vi "MAIN_green.vi"() -> ()   [LabVIEW 2011]
uses:
  <vilib>/userDefined/High Color/IMAQdx.ctl
  <vilib>/vision/driver/NI_Vision_Acquisition_Software.lvlib
  <vilib>/vision/NI_Vision_Development_Module.lvlib
panel:
  out "error out 6":errorcluster
  out "error out 5":errorcluster
  out "error out 4":errorcluster
  in  "SLM 2":enum32{"Viewer & Positioner", "Hologram Loader"}(tab)
  out "<< CGH_y\n      SLM 2":T1(plugin-control)
  in  "X position 2":dbl(slide)=1.056105610561056 scale=0.0..10.0
  in  "Fine:":dbl(slide)=2.7960526315789473 scale=0.0..10.0
  out "X 2":dbl
  in  "Fine:":dbl(slide)=4.922480620155039 scale=0.0..10.0
  in  "Y position 3":dbl(slide)=3.875968992248062 scale=0.0..10.0
  out "Y position 2":dbl
  out "String 2":string
  out "String 3":string
  out "SLM 3":T1(plugin-control)
  in  "Radio Buttons":T2(radio)=enum."Radio Selection 2"
  in  "Semi2":bool caption="Boolean"
  in  "Phase correction 2":bool
  in  "M4":bool
  in  "Holo:":dbl=1.0
  out "Ph2 2":dbl
  out "[0 255]":dbl
  out "Ph2":dbl
  in  "Phase:":dbl(slide) scale=0.0..360.0
  out "T2":dbl=100.0
  in  "Trans.:":dbl(slide)=100.0 scale=0.0..100.0
  in  "Active SLM2":bool=TRUE
  in  "SLM 1":enum32{"Viewer & Positioner", "Hologram Loader"}(tab)
  out "CGH_x >>\nSLM 1":T1(plugin-control)
  in  "Y position":dbl(slide)=3.292682926829268 scale=0.0..10.0
  in  "X position 1":dbl(slide)=8.30670926517572 scale=0.0..10.0
  in  "Fine:":dbl(slide)=7.667731629392971 scale=0.0..10.0
  in  "Fine:":dbl(slide)=0.7636363636363636 scale=0.0..10.0
  out "X position":dbl
  out "Y position 1":dbl
  out "String":string
  in  "Radio Buttons 2":T2(radio)=enum."Radio Selection 2"
  in  "Semi":bool caption="Boolean"
  in  "Phase correction":bool caption="Amplitude correction"
  in  "M4 2":bool caption="Amplitude correction"
  in  "Holo:":dbl=1.0
  out "Ph1 2":dbl
  out "[0 255]":dbl
  out "Ph1":dbl
  in  "Phase:":dbl(slide) scale=0.0..360.0
  out "T1":dbl=100.0
  in  "Trans.:":dbl(slide)=100.0 scale=0.0..100.0
  out "SLM 2":T1(plugin-control)
  in  "Active SLM1":bool=TRUE
  out "String 4":string
  in  "Parada Total":bool
  in  "Tab Control":enum32{"Laser Control", "CCD viewer"}(tab)
  in  "APTLaser":refnum<k7>(container) caption="Resume"
  in  "LaserON":bool
  in  "Set Current at:":sgl=70.0 caption="mA"
  out "Color Box":u32(colorbox)
  out "Power":dbl(knob) caption="mW" scale=0.0..16.0
  in  "Save":bool
  in  "Focused":bool
  out "Image":T1(plugin-control)
  out "Histograph":T3(graph)={"Starting Value"=-32768.0, "Incremental Value"=1.0, "Histogram"=array[65536 elements]}
  out "# Sat. Pixels":sgl(slide) scale=0.0..5000.0
  out "error out 3":errorcluster
  out "error out 2":errorcluster
  out "error out":errorcluster
  out "path":path
  out "selected path 2":path
  out "selected path":path
  # "Arbitrary value settings:"
  # "For gray levels ->"
  # "%"
  # "º"
  # "\\pi rad"
  # "Arbitrary value settings:"
  # "For gray levels ->"
  # "%"
  # "º"
  # "\\pi rad"
  # "Paraxial"
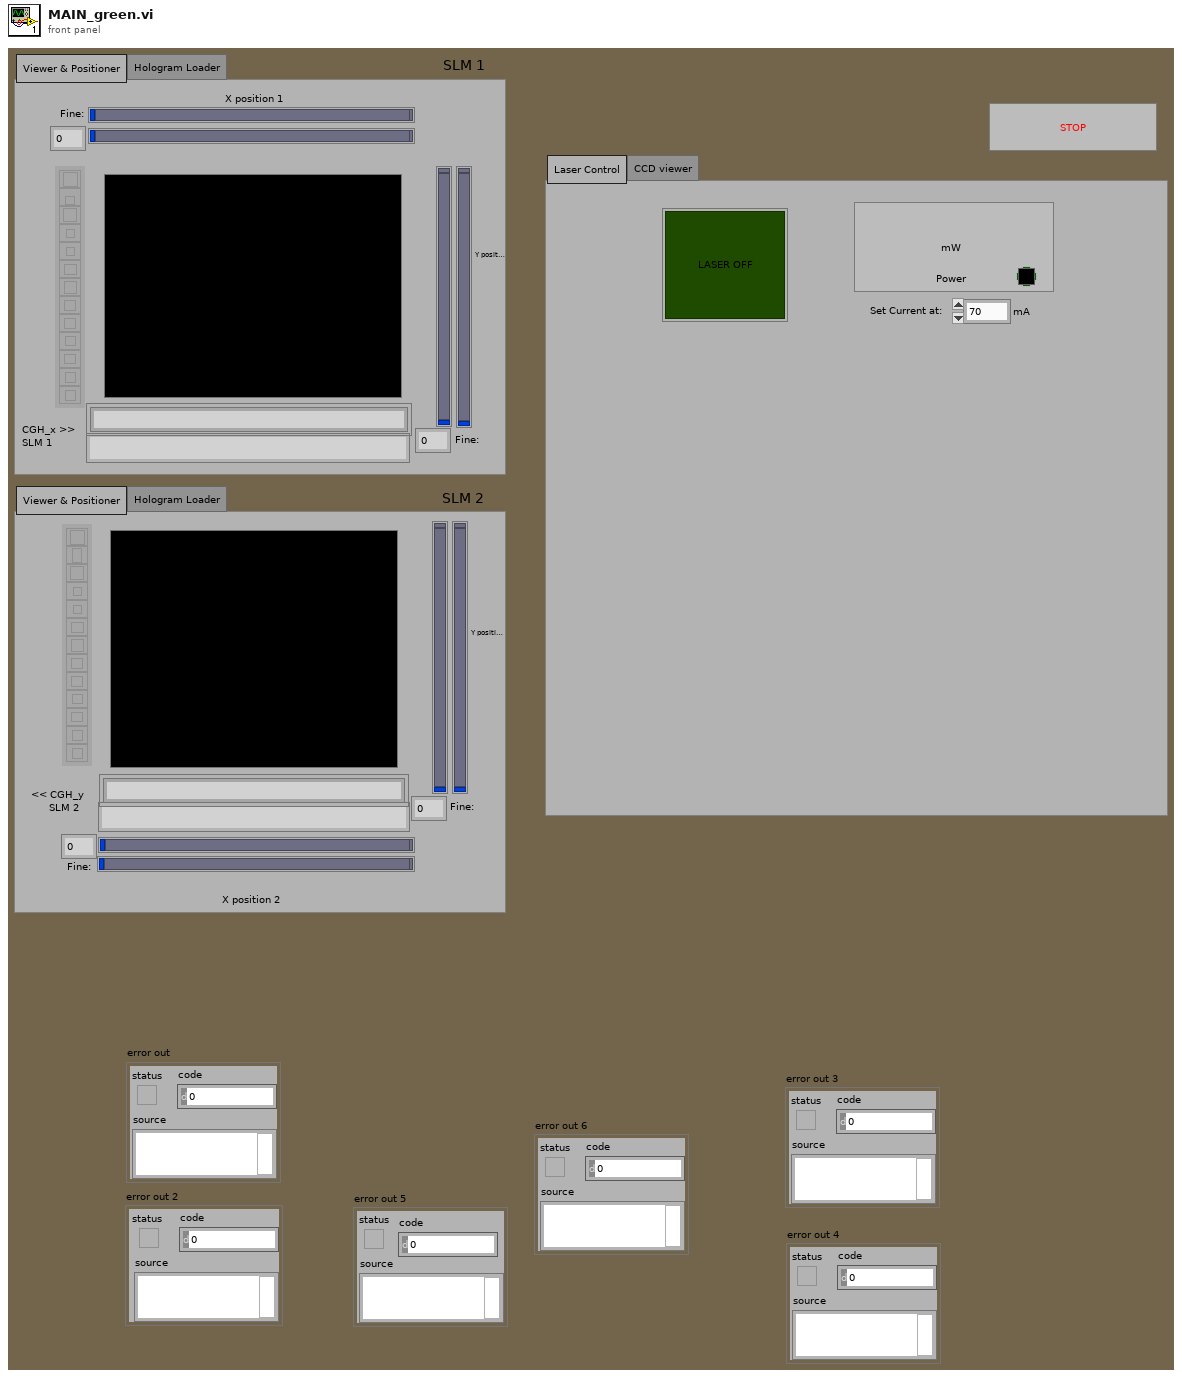
[diagram p1: front panel]
types:
  T1 = typedef "IMAQ Image.ctl" = refnum<image>
  T2 = enum32{"Radio Selection 1", "Radio Selection 2", "Radio Selection 3", "Radio Selection 4", "Radio Selection 5", "Radio Selection 6", "Radio Selection 7"}
  T3 = cluster{"Starting Value":sgl, "Incremental Value":sgl, "Histogram":u32[]}
  T4 = typedef "IMAQdx.ctl" = refnum<k21>
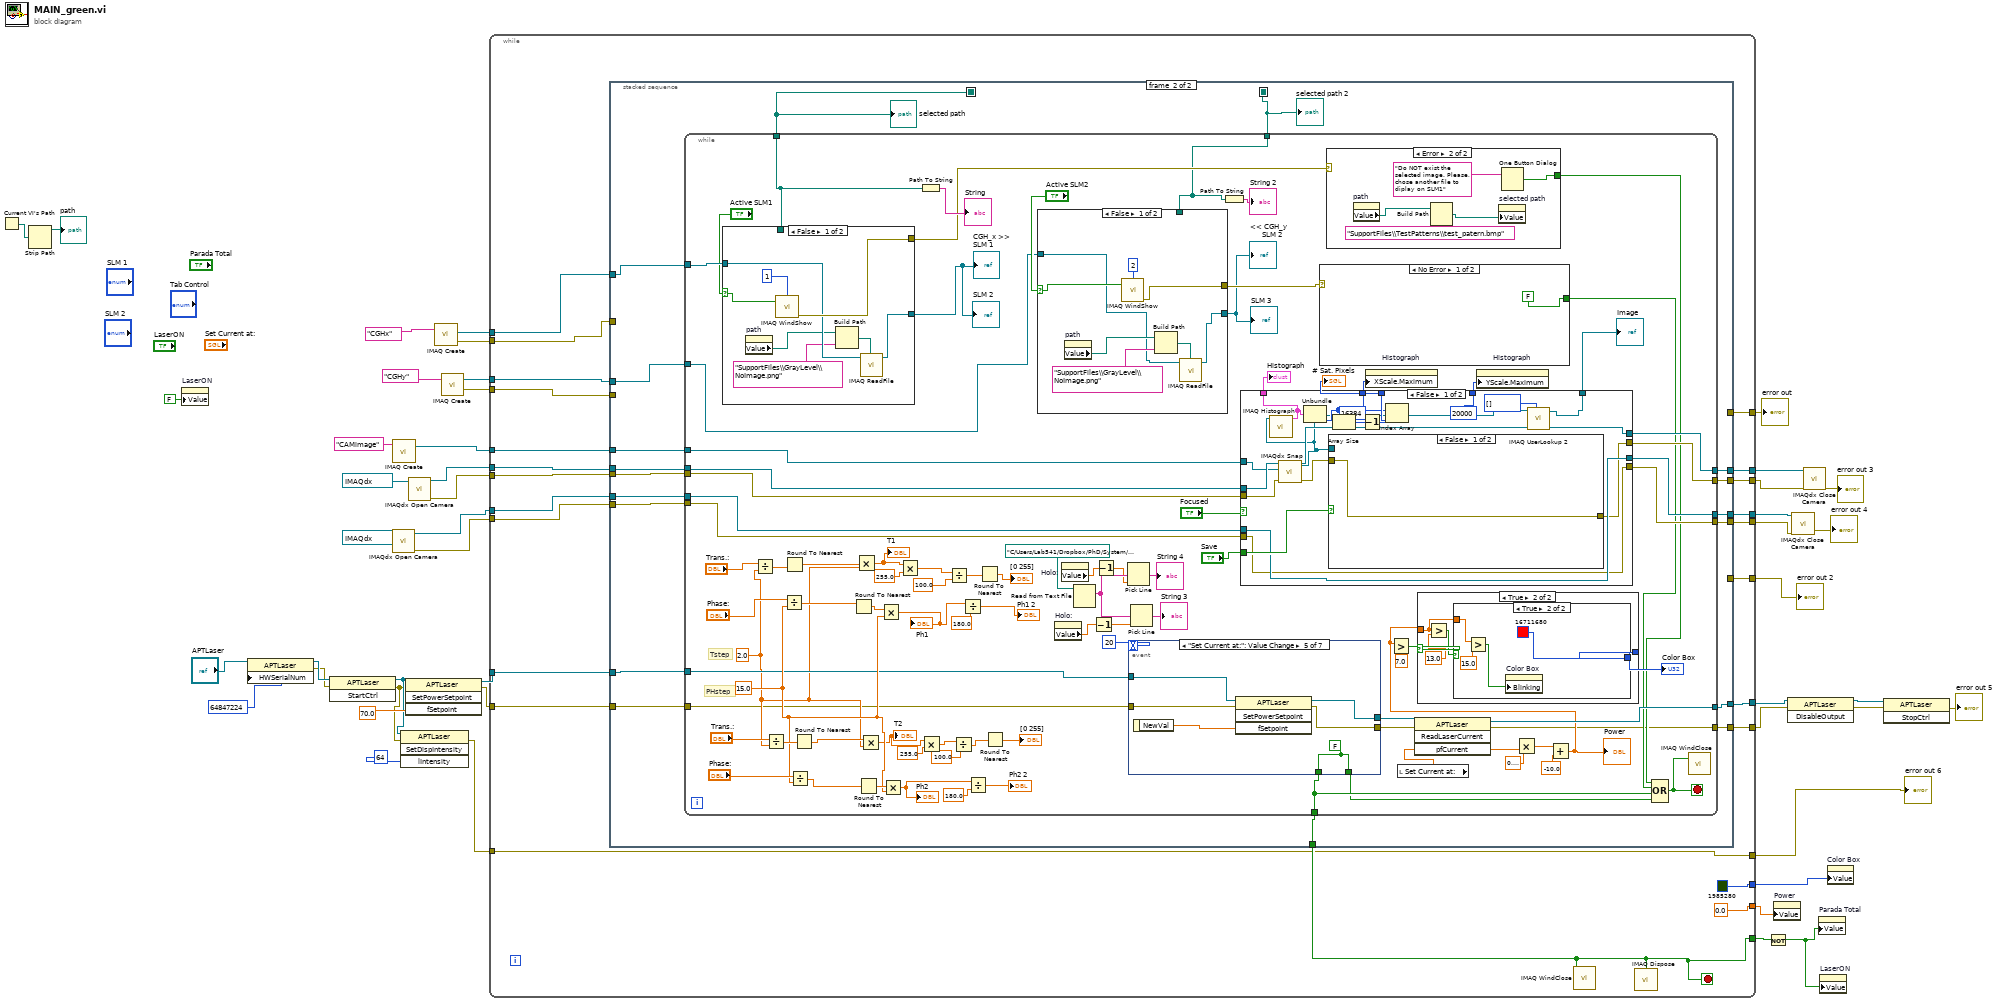
[diagram p0: block diagram]
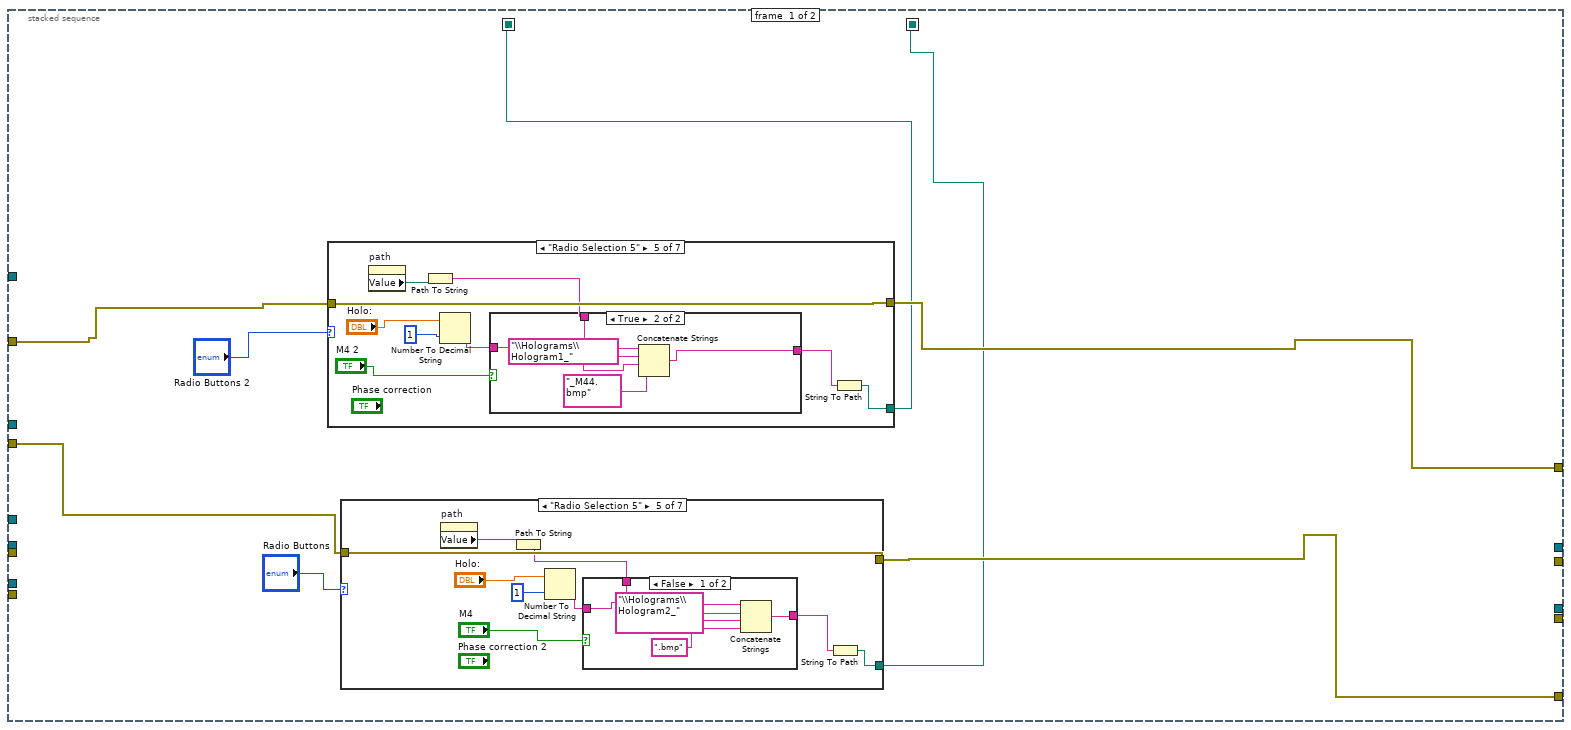
[diagram p2: hidden frame]
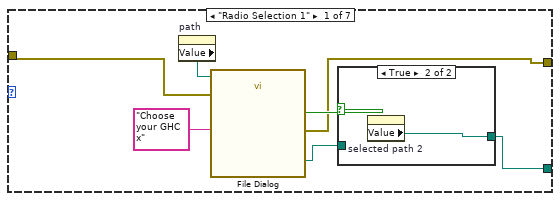
[diagram p3: hidden frame]
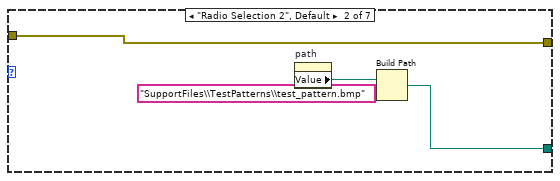
[diagram p5: hidden frame]
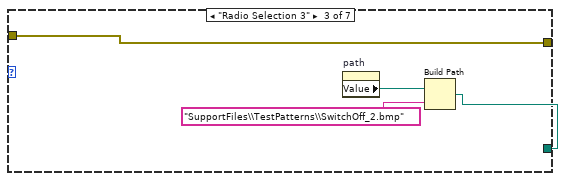
[diagram p6: hidden frame]
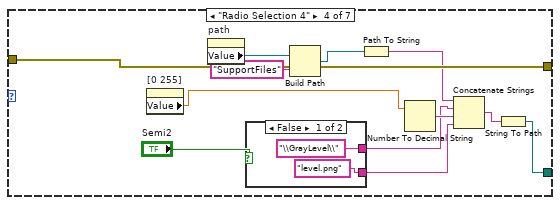
[diagram p7: hidden frame]
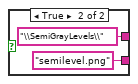
[diagram p8: hidden frame]
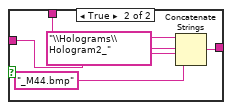
[diagram p9: hidden frame]
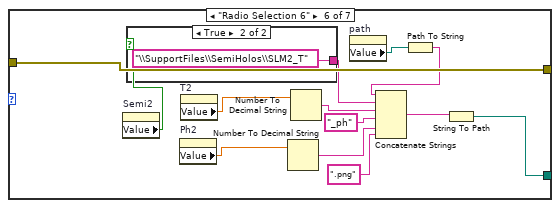
[diagram p10: hidden frame]
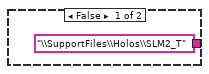
[diagram p11: hidden frame]
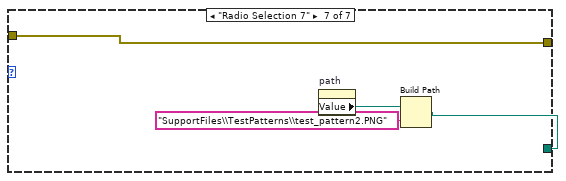
[diagram p12: hidden frame]
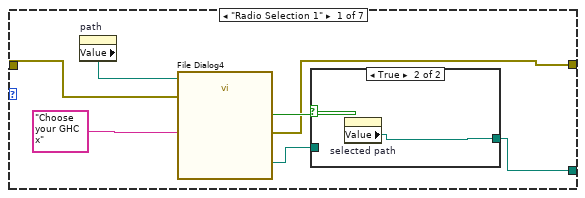
[diagram p13: hidden frame]
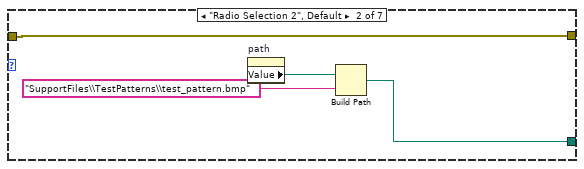
[diagram p15: hidden frame]
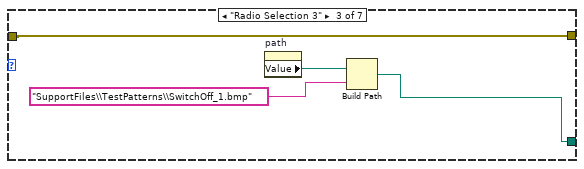
[diagram p16: hidden frame]
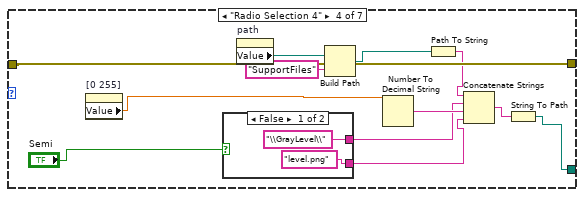
[diagram p17: hidden frame]
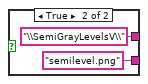
[diagram p18: hidden frame]
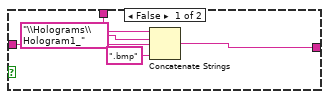
[diagram p19: hidden frame]
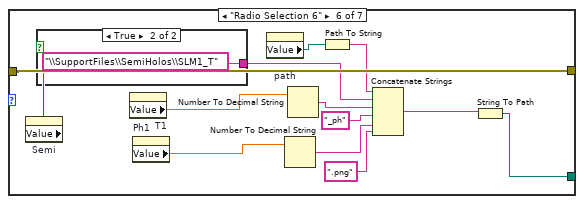
[diagram p20: hidden frame]
diagram:
  n1 = Current VI's Path() -> (path=w40:path)
  n2 = Strip Path(path=w40) -> (stripped path=→"path":path)  [unwired: 1 out]
  n3 = property on="LaserON" class="Bool (strict)"("Value"=FALSE ("LaserON")) -> ()  [unwired: 2 in, 2 out]
  n4 = property class="APTLaser"(reference="APTLaser", "HWSerialNum"=64847224) -> (reference out=w30:refnum<k7>, error out=w8:errorcluster)  [unwired: 1 in]
  n5 = invoke class="APTLaser" method="StartCtrl"(reference=w30, error in=w8) -> (reference out=w19:refnum<k7>, error out=w3:errorcluster)  [unwired: 1 in, 1 out]
  n6 = call <vilib>:"IMAQdx Open Camera.vi"("Session In"=T4 "Focused") -> ("error out"=w12:errorcluster, "Session Out"=w11:T4)  [unwired: 9 in]
  n7 = call "IMAQ Create"("Image Name"="CAMimage") -> ("New Image"=w36:T1)  [unwired: 4 in, 1 out]
  n8 = invoke class="APTLaser" method="SetDispIntensity"(reference=w19, error in=w3, "lIntensity"=64) -> (error out=w2:errorcluster)  [unwired: 1 in, 3 out]
  n9 = invoke class="APTLaser" method="SetPowerSetpoint"(reference=w19, error in=w3, "fSetpoint"=sgl 70.0) -> (reference out=w25:refnum<k7>, error out=w7:errorcluster)  [unwired: 1 in, 2 out]
  n10 = call <vilib>:"IMAQdx Open Camera.vi"("Session In"=T4 "Paraxial") -> ("error out"=w10:errorcluster, "Session Out"=w9:T4)  [unwired: 9 in]
  n11 = call "IMAQ Create"("Image Name"="CGHx") -> ("New Image"=w44:T1, "error out"=w41:errorcluster)  [unwired: 4 in]
  n12 = call "IMAQ Create"("Image Name"="CGHy") -> ("New Image"=w43:T1, "error out"=w42:errorcluster)  [unwired: 4 in]
  n13 = while {
    tunnel: w44 -> [w69]
    tunnel: w43 -> [w68]
    tunnel: w42 -> [w67]
    tunnel: [w66] -> w32
    tunnel: w41 -> [w65]
    tunnel: [w64] -> w33
    tunnel: [w50] -> w38
    tunnel: w36 -> [w63]
    tunnel: w9 -> [w62]
    tunnel: w10 -> [w61]
    tunnel: w11 -> [w60]
    tunnel: w12 -> [w59]
    tunnel: [w58] -> w28
    tunnel: w25 -> [w57]
    tunnel: [0.0 ("Power")] -> w21
    tunnel: [u32 1985280] -> w22
    tunnel: [w54] -> w16
    tunnel: [w53] -> w15
    tunnel: [w52] -> w14
    tunnel: [w51] -> w13
    tunnel: w7 -> [w49]
    tunnel: [w48] -> w6
    tunnel: w2 -> [w47]
    tunnel: [w47] -> w1
    stop <- w50 stop-if-true
    n14 = stacked-sequence {
      seq-local: [w73 _] -> [_ w224]
      seq-local: [w72 _] -> [_ w223]
      tunnel: w69 -> [_ w236]
      tunnel: w68 -> [_ w237]
      tunnel: [_ w222] -> w50
      tunnel: w67 -> [w71 _]
      tunnel: [w77 _] -> w66
      tunnel: w65 -> [w76 _]
      tunnel: [w75 _] -> w64
      tunnel: w63 -> [_ w235]
      tunnel: w62 -> [_ w234]
      tunnel: w61 -> [_ w233]
      tunnel: w60 -> [_ w232]
      tunnel: w59 -> [_ w231]
      tunnel: w57 -> [_ w230]
      tunnel: [_ w229] -> w58
      tunnel: [_ w228] -> w54
      tunnel: [_ w227] -> w53
      tunnel: [_ w226] -> w52
      tunnel: [_ w225] -> w51
      tunnel: w49 -> [_ w221]
      tunnel: [_ w220] -> w48
      frame #0 {
        n15 = case shown="\"Radio Selection 5\"" "Radio Buttons 2" {
          tunnel: w76 -> [w151 w161 w165 w177 w190 w213 w219]
          tunnel: [w150 w158 w162 w174 w188 w207 w216] -> w73
          tunnel: [w152 w161 w165 w177 w190 w213 w219] -> w75
          frame "Radio Selection 1" {
            n16 = property on="path" class="Path"() -> ("Value"=w149:path)  [unwired: 2 in, 2 out]
            n17 = call "File Dialog4"("start path"=w149, "prompt"="Choose your GHC x", "error in"=w151) -> ("selected path"=w154:path, "cancelled"=w153:bool, "error out"=w152:errorcluster)  [unwired: 9 in, 1 out]
            n18 = case shown="True" w153 {
              tunnel: [w156 w157] -> w150
              tunnel: w154 -> [w156 _]
              frame False {
              }
              frame True {
                n19 = property on="selected path" class="Path"() -> ("Value"=w157:path)  [unwired: 2 in, 2 out]
              }
            }
          }
          frame "Radio Selection 2", Default {
            n20 = property on="path" class="Path"() -> ("Value"=w160:path)  [unwired: 2 in, 2 out]
            n21 = Build Path(base path=w160, name or relative path="SupportFiles\\TestPatterns\\test_pattern.bmp") -> (appended path=w158:path)
          }
          frame "Radio Selection 3" {
            n22 = property on="path" class="Path"() -> ("Value"=w164:path)  [unwired: 2 in, 2 out]
            n23 = Build Path(base path=w164, name or relative path="SupportFiles\\TestPatterns\\SwitchOff_1.bmp") -> (appended path=w162:path)
          }
          frame "Radio Selection 4" {
            n24 = property on="[0 255]" class="DigNum (strict)"() -> ("Value"=w166:dbl)  [unwired: 2 in, 2 out]
            n25 = case shown="False" "Semi" {
              tunnel: ["\\GrayLevel\\" ("name or relative path") "\\SemiGrayLevelsV\\" ("name or relative path")] -> w168
              tunnel: ["level.png" ("string") "semilevel.png" ("string")] -> w167
              frame False {
              }
              frame True {
              }
            }
            n26 = property on="path" class="Path"() -> ("Value"=w173:path)  [unwired: 2 in, 2 out]
            n27 = Build Path(base path=w173, name or relative path="SupportFiles") -> (appended path=w171:path)
            n28 = Number To Decimal String(number=w166) -> (decimal integer string=w176:string)  [unwired: 1 in]
            n29 = Path To String(path=w171) -> (string=w170:string)
            n30 = Concatenate Strings(w170, w168, w176, w167) -> (w175:string)
            n31 = String To Path(string=w175) -> (path=w174:path)
          }
          frame "Radio Selection 5" {
            n32 = property on="path" class="Path"() -> ("Value"=w184:path)  [unwired: 2 in, 2 out]
            n33 = Path To String(path=w184) -> (string=w183:string)
            n34 = Number To Decimal String(number="Holo:", width (-)=i16 1) -> (decimal integer string=w186:string)
            n35 = case shown="True" "M4 2" {
              tunnel: [w194 w198] -> w189
              tunnel: w186 -> [w193 w197]
              tunnel: w183 -> [w192 w196]
              frame False {
                n36 = Concatenate Strings(w192, "\\Holograms\\Hologram1_" ("string"), w193, ".bmp" ("string")) -> (w194:string)
              }
              frame True {
                n37 = Concatenate Strings(w196, "\\Holograms\\Hologram1_" ("string"), w197, "_M44.bmp" ("string")) -> (w198:string)
              }
            }
            n38 = String To Path(string=w189) -> (path=w188:path)
          }
          frame "Radio Selection 6" {
            n39 = property on="Semi" class="Bool (strict)"() -> ("Value"=w201:bool)  [unwired: 2 in, 2 out]
            n40 = case shown="True" w201 {
              tunnel: ["\\SupportFiles\\Holos\\SLM1_T" ("name or relative path") "\\SupportFiles\\SemiHolos\\SLM1_T" ("name or relative path")] -> w202
              frame False {
              }
              frame True {
              }
            }
            n41 = property on="T1" class="DigNum (strict)"() -> ("Value"=w206:dbl)  [unwired: 2 in, 2 out]
            n42 = property on="Ph1" class="DigNum (strict)"() -> ("Value"=w205:dbl)  [unwired: 2 in, 2 out]
            n43 = property on="path" class="Path"() -> ("Value"=w204:path)  [unwired: 2 in, 2 out]
            n44 = Number To Decimal String(number=w205) -> (decimal integer string=w211:string)  [unwired: 1 in]
            n45 = Number To Decimal String(number=w206) -> (decimal integer string=w212:string)  [unwired: 1 in]
            n46 = Path To String(path=w204) -> (string=w203:string)
            n47 = Concatenate Strings(w203, w202, w212, "_ph" ("Master Thesis (folder)"), w211, ".png" ("Master Thesis (folder)")) -> (w208:string)
            n48 = String To Path(string=w208) -> (path=w207:path)
          }
          frame "Radio Selection 7" {
            n49 = property on="path" class="Path"() -> ("Value"=w218:path)  [unwired: 2 in, 2 out]
            n50 = Build Path(base path=w218, name or relative path="SupportFiles\\TestPatterns\\test_pattern2V.PNG") -> (appended path=w216:path)
          }
        }
        n51 = case shown="\"Radio Selection 5\"" "Radio Buttons" {
          tunnel: w71 -> [w80 w90 w94 w106 w119 w142 w148]
          tunnel: [w79 w87 w91 w103 w117 w136 w145] -> w72
          tunnel: [w81 w90 w94 w106 w119 w142 w148] -> w77
          frame "Radio Selection 1" {
            n52 = property on="path" class="Path"() -> ("Value"=w78:path)  [unwired: 2 in, 2 out]
            n53 = call "File Dialog"("start path"=w78, "prompt"="Choose your GHC x", "error in"=w80) -> ("selected path"=w83:path, "cancelled"=w82:bool, "error out"=w81:errorcluster)  [unwired: 9 in, 1 out]
            n54 = case shown="True" w82 {
              tunnel: [w85 w86] -> w79
              tunnel: w83 -> [w85 _]
              frame False {
              }
              frame True {
                n55 = property on="selected path 2" class="Path"() -> ("Value"=w86:path)  [unwired: 2 in, 2 out]
              }
            }
          }
          frame "Radio Selection 2", Default {
            n56 = property on="path" class="Path"() -> ("Value"=w89:path)  [unwired: 2 in, 2 out]
            n57 = Build Path(base path=w89, name or relative path="SupportFiles\\TestPatterns\\test_pattern.bmp") -> (appended path=w87:path)
          }
          frame "Radio Selection 3" {
            n58 = property on="path" class="Path"() -> ("Value"=w93:path)  [unwired: 2 in, 2 out]
            n59 = Build Path(base path=w93, name or relative path="SupportFiles\\TestPatterns\\SwitchOff_2.bmp") -> (appended path=w91:path)
          }
          frame "Radio Selection 4" {
            n60 = property on="[0 255]" class="DigNum (strict)"() -> ("Value"=w95:dbl)  [unwired: 2 in, 2 out]
            n61 = property on="path" class="Path"() -> ("Value"=w102:path)  [unwired: 2 in, 2 out]
            n62 = case shown="False" "Semi2" {
              tunnel: ["\\GrayLevel\\" ("name or relative path") "\\SemiGrayLevels\\" ("name or relative path")] -> w98
              tunnel: ["level.png" ("string") "semilevel.png" ("string")] -> w97
              frame False {
              }
              frame True {
              }
            }
            n63 = Build Path(base path=w102, name or relative path="SupportFiles") -> (appended path=w100:path)
            n64 = Path To String(path=w100) -> (string=w99:string)
            n65 = Number To Decimal String(number=w95) -> (decimal integer string=w105:string)  [unwired: 1 in]
            n66 = Concatenate Strings(w99, w98, w105, w97) -> (w104:string)
            n67 = String To Path(string=w104) -> (path=w103:path)
          }
          frame "Radio Selection 5" {
            n68 = property on="path" class="Path"() -> ("Value"=w114:path)  [unwired: 2 in, 2 out]
            n69 = Path To String(path=w114) -> (string=w113:string)
            n70 = Number To Decimal String(number="Holo:", width (-)=i16 1) -> (decimal integer string=w112:string)
            n71 = case shown="False" "M4" {
              tunnel: w113 -> [w122 w129]
              tunnel: [w120 w126] -> w118
              tunnel: w112 -> [w123 w127]
              frame False {
                n72 = Concatenate Strings(w122, "\\Holograms\\Hologram2_" ("string"), w123, ".bmp" ("string")) -> (w120:string)
              }
              frame True {
                n73 = Concatenate Strings(w129, "\\Holograms\\Hologram2_" ("string"), w127, "_M44.bmp" ("string")) -> (w126:string)
              }
            }
            n74 = String To Path(string=w118) -> (path=w117:path)
          }
          frame "Radio Selection 6" {
            n75 = property on="Semi2" class="Bool (strict)"() -> ("Value"=w133:bool)  [unwired: 2 in, 2 out]
            n76 = case shown="True" w133 {
              tunnel: ["\\SupportFiles\\Holos\\SLM2_T" ("name or relative path") "\\SupportFiles\\SemiHolos\\SLM2_T" ("name or relative path")] -> w130
              frame False {
              }
              frame True {
              }
            }
            n77 = property on="Ph2" class="DigNum (strict)"() -> ("Value"=w134:dbl)  [unwired: 2 in, 2 out]
            n78 = property on="T2" class="DigNum (strict)"() -> ("Value"=w135:dbl)  [unwired: 2 in, 2 out]
            n79 = Number To Decimal String(number=w134) -> (decimal integer string=w140:string)  [unwired: 1 in]
            n80 = Number To Decimal String(number=w135) -> (decimal integer string=w141:string)  [unwired: 1 in]
            n81 = property on="path" class="Path"() -> ("Value"=w132:path)  [unwired: 2 in, 2 out]
            n82 = Path To String(path=w132) -> (string=w131:string)
            n83 = Concatenate Strings(w131, w130, w141, "_ph" ("Master Thesis (folder)"), w140, ".png" ("Master Thesis (folder)")) -> (w137:string)
            n84 = String To Path(string=w137) -> (path=w136:path)
          }
          frame "Radio Selection 7" {
            n85 = property on="path" class="Path"() -> ("Value"=w147:path)  [unwired: 2 in, 2 out]
            n86 = Build Path(base path=w147, name or relative path="SupportFiles\\TestPatterns\\test_pattern2.PNG") -> (appended path=w145:path)
          }
        }
      }
      frame #1 {
        n87 = while {
          tunnel: [w260] -> w222
          tunnel: w224 -> [w319]
          tunnel: w223 -> [w256]
          tunnel: w237 -> [w261]
          tunnel: w236 -> [w326]
          tunnel: w235 -> [w293]
          tunnel: w234 -> [w292]
          tunnel: w233 -> [w291]
          tunnel: w232 -> [w290]
          tunnel: w231 -> [w289]
          tunnel: [w280] -> w229
          tunnel: w230 -> [w283]
          tunnel: [w270] -> w228
          tunnel: [w269] -> w227
          tunnel: [w268] -> w226
          tunnel: [w267] -> w225
          tunnel: w221 -> [w248]
          tunnel: [w246] -> w220
          stop <- w294 stop-if-true
          w299 = 15.0 ("x")
          w274 = 2.0 ("x")
          # "PHstep"
          # "Tstep"
          n88 = case shown="False" "Active SLM1" {
            selector: "Active SLM1" -> [w352 _]
            tunnel: w326 -> [w351 w368]
            tunnel: w319 -> [_ w364]
            tunnel: [w350 w363] -> w255
            tunnel: [w353 w362] -> w262
            frame False {
              n89 = property on="path" class="Path"() -> ("Value"=w348:path)  [unwired: 2 in, 2 out]
              n90 = call "IMAQ WindShow"("Hide/Show (Show)"=w352, "Window Number (0...15)"=1) -> ("error out"=w353:errorcluster)  [unwired: 4 in, 2 out]
              n91 = Build Path(base path=w348, name or relative path="SupportFiles\\GrayLevel\\NoImage.png") -> (appended path=w349:path)
              n92 = call "IMAQ ReadFile"("File Path"=w349, "Image"=w351) -> ("Image Out"=w350:T1)  [unwired: 5 in, 4 out]
            }
            frame True {
              n93 = Multiply(x="X position 1", y=1.0 ("x")) -> (x*y=w361:dbl)
              n94 = call "IMAQ ReadFile"("File Path"=w364, "Image"=w368) -> ("error out"=w362:errorcluster, "Image Out"=w360:T1)  [unwired: 5 in, 3 out]
              n95 = call "WinPositioner.vi"("Image"=w360, "X position"=w361, "Fine X position"="Fine:", "Y position"="Y position", "Fine Y position"="Fine:", "Display?"=TRUE) -> ("CGH_x"=w363:T1, "X position"=→"X position":dbl, "Y position"=→"Y position 1":dbl)  [unwired: 2 in]
            }
          }
          "CGH_x >>\nSLM 1" <- w255
          "SLM 2" <- w255
          n96 = Divide(x="Trans.:", y=w274) -> (x/y=w318:dbl)
          n97 = Divide(x="Trans.:", y=w274) -> (x/y=w310:dbl)
          n98 = Divide(x="Phase:", y=w299) -> (x/y=w325:dbl)
          n99 = Round To Nearest(number=w318) -> (nearest integer value=w322:dbl)
          n100 = Divide(x="Phase:", y=w299) -> (x/y=w301:dbl)
          n101 = Round To Nearest(number=w310) -> (nearest integer value=w309:dbl)
          n102 = Round To Nearest(number=w325) -> (nearest integer value=w323:dbl)
          n103 = Multiply(x=w322, y=w274) -> (x*y=w317:dbl)
          "T1" <- w317
          n104 = Round To Nearest(number=w301) -> (nearest integer value=w300:dbl)
          n105 = Multiply(x=w309, y=w274) -> (x*y=w298:dbl)
          "T2" <- w298
          n106 = Multiply(x=w323, y=w299) -> (x*y=w311:dbl)
          "Ph1" <- w311
          n107 = Multiply(x=w300, y=w299) -> (x*y=w297:dbl)
          "Ph2" <- w297
          n108 = Multiply(x=w317, y=255.0) -> (x*y=w315:dbl)
          n109 = Path To String(path=w319) -> (string=→"String":string)
          n110 = Multiply(x=w298, y=255.0) -> (x*y=w307:dbl)
          n111 = Divide(x=w315, y=100.0) -> (x/y=w312:dbl)
          n112 = Divide(x=w307, y=100.0) -> (x/y=w305:dbl)
          n113 = Divide(x=w311, y=180.0) -> (x/y=→"Ph1 2":dbl)
          n114 = Divide(x=w297, y=180.0) -> (x/y=→"Ph2 2":dbl)
          n115 = Round To Nearest(number=w312) -> (nearest integer value=→"[0 255]":dbl)
          n116 = Round To Nearest(number=w305) -> (nearest integer value=→"[0 255]":dbl)
          n117 = case shown="False" "Active SLM2" {
            selector: "Active SLM2" -> [w332 _]
            tunnel: w261 -> [w327 w345]
            tunnel: [w328 w342] -> w254
            tunnel: w256 -> [_ w335]
            tunnel: [w334 w344] -> w264
            frame False {
              n118 = property on="path" class="Path"() -> ("Value"=w330:path)  [unwired: 2 in, 2 out]
              n119 = call "IMAQ WindShow"("Hide/Show (Show)"=w332, "Window Number (0...15)"=2) -> ("error out"=w334:errorcluster)  [unwired: 4 in, 2 out]
              n120 = Build Path(base path=w330, name or relative path="SupportFiles\\GrayLevel\\NoImage.png") -> (appended path=w331:path)
              n121 = call "IMAQ ReadFile"("File Path"=w331, "Image"=w327) -> ("Image Out"=w328:T1)  [unwired: 5 in, 4 out]
            }
            frame True {
              n122 = call "IMAQ ReadFile"("File Path"=w335, "Image"=w345) -> ("error out"=w344:errorcluster, "Image Out"=w343:T1)  [unwired: 5 in, 3 out]
              n123 = call "WinPositioner.vi"("Image"=w343, "X position"="X position 2", "Fine X position"="Fine:", "Y position"="Y position 3", "Fine Y position"="Fine:", "Display?"=FALSE) -> ("CGH_x"=w342:T1, "X position"=→"X 2":dbl, "Y position"=→"Y position 2":dbl)  [unwired: 2 in]
            }
          }
          "<< CGH_y\n      SLM 2" <- w254
          "SLM 3" <- w254
          n124 = property on="Holo:" class="DigNum (strict)"() -> ("Value"=w241:dbl)  [unwired: 2 in, 2 out]
          n125 = property on="Holo:" class="DigNum (strict)"() -> ("Value"=w243:dbl)  [unwired: 2 in, 2 out]
          n126 = Read from Text File(file (use dialog)=path "C:/Users/Lab541/Dropbox/PhD/System/+scripts/design_kinds.txt") -> (text=w244:string)  [unwired: 3 in, 3 out]
          n127 = Decrement(x=w241) -> (x-1=w240:dbl)
          n128 = Decrement(x=w243) -> (x-1=w242:dbl)
          n129 = Pick Line(multi-line string=w244, line index=w242) -> (output string=→"String 4":string)  [unwired: 1 in]
          n130 = event shown="[4] \"Set Current at:\": Value Change" {
            selector: _ -> [_ _ _ _ _ _ _]
            dyn-events: _ -> [_ _ _ _ _ _ _]
            timeout: 20 -> [_ _ _ _ _ _ _]
            tunnel: [w389 w400 w404 w408 w412 w417 w422] -> w281
            tunnel: w283 -> [w387 w400 w404 w408 w413 w417 w422]
            tunnel: [w386 w399 TRUE ("value") TRUE ("value") w411 w416 w421] -> w259
            tunnel: [w386 w399 w402 FALSE ("NewVal") w411 w416 w421] -> w260
            tunnel: w248 -> [w385 w398 w401 w405 w410 w415 w420]
            tunnel: [w384 w398 w401 w405 w409 w415 w420] -> w247
            event "LaserON": Value Change {
              w386 = FALSE ("NewVal")
              n131 = event-data() -> ("NewVal"=w388:bool)  [unwired: 1 in]
              n132 = case shown="True" w388 {
                tunnel: [w393 w397] -> w389
                tunnel: w387 -> [w392 w396]
                tunnel: w385 -> [w391 w395]
                tunnel: [w390 w394] -> w384
                frame False {
                  n133 = invoke class="APTLaser" method="DisableOutput"(reference=w392, error in=w391) -> (reference out=w393:refnum<k7>, error out=w390:errorcluster)  [unwired: 1 in, 1 out]
                }
                frame True {
                  n134 = invoke class="APTLaser" method="EnableOutput"(reference=w396, error in=w395) -> (reference out=w397:refnum<k7>, error out=w394:errorcluster)  [unwired: 1 in, 1 out]
                }
              }
            }
            event Timeout {
              w399 = FALSE ("NewVal")
              n135 = event-data() -> ()  [unwired: 1 in, 2 out]
            }
            event "Parada Total": Value Change {
              n136 = event-data() -> ("NewVal"=w402:bool)  [unwired: 1 in]
            }
            event "Radio Buttons", "Radio Buttons 2", "Holo:", "Holo:", "M4", "M4 2", "Phase correction", "Phase correction 2", "Semi", "Semi2": Value Change; "Trans.:", "Phase:", "Trans.:", "Phase:": Mouse Up {
              n137 = event-data() -> ()  [unwired: 1 in, 4 out]
            }
            event "Set Current at:": Value Change {
              w411 = FALSE ("value")
              n138 = event-data() -> ("NewVal"=w414:sgl)  [unwired: 1 in]
              n139 = invoke class="APTLaser" method="SetPowerSetpoint"(reference=w413, error in=w410, "fSetpoint"=w414) -> (reference out=w412:refnum<k7>, error out=w409:errorcluster)  [unwired: 1 in, 2 out]
            }
            event "Active SLM1": Value Change {
              w416 = FALSE ("NewVal")
              n140 = event-data() -> ("NewVal"=w419:bool)  [unwired: 1 in]
              n141 = call "IMAQ WindShow"("Hide/Show (Show)"=w419, "Window Number (0...15)"=1) -> ()  [unwired: 4 in, 3 out]
            }
            event "Active SLM2": Value Change {
              w421 = FALSE ("NewVal")
              n142 = event-data() -> ("NewVal"=w423:bool)  [unwired: 1 in]
              n143 = call "IMAQ WindShow"("Hide/Show (Show)"=w423, "Window Number (0...15)"=2) -> ()  [unwired: 4 in, 3 out]
            }
          }
          n144 = Pick Line(multi-line string=w244, line index=w240) -> (output string=→"String 3":string)  [unwired: 1 in]
          n145 = Path To String(path=w256) -> (string=→"String 2":string)
          n146 = case shown="False" "Focused" {
            tunnel: "Save" -> [w441 w473]
            tunnel: [w439 w476] -> w267
            tunnel: [w426 w467] -> w253
            tunnel: w293 -> [w435 w471]
            tunnel: w292 -> [w437 w469]
            tunnel: w291 -> [w436 w468]
            tunnel: w290 -> [w440 w470]
            tunnel: w289 -> [w439 w472]
            tunnel: [w440 w474] -> w268
            tunnel: [w442 w469] -> w270
            tunnel: [w438 w468] -> w269
            tunnel: [w434 w463] -> w252
            tunnel: [w433 w462] -> w251
            tunnel: [16384 768] -> w250
            tunnel: [20000 200000] -> w249
            frame False {
              n147 = call <vilib>:"IMAQdx Snap.vi"("error in"=w436, "Image In"=w435, "Session In"=w437) -> ("error out"=w443:errorcluster, "Image Out"=w427:T1, "Session Out"=w442:T4)  [unwired: 6 in]
              n148 = call "IMAQ Histograph"("Image"=w427) -> ("Histogram Graph"=w434:T3)  [unwired: 7 in, 3 out]
              n149 = Unbundle(w434) -> ("Histogram"=w432:u32[])  [unwired: 2 out]
              n150 = case shown="False" w441 {
                tunnel: [w444 w447] -> w438
                tunnel: w427 -> [_ w445]
                tunnel: w443 -> [w444 w446]
                frame False {
                }
                frame True {
                  n151 = property on="path" class="Path"() -> ("Value"=w455:path)  [unwired: 2 in, 2 out]
                  n152 = Build Path(base path=w455, name or relative path="Images") -> (appended path=w454:path)
                  n153 = call "File Dialog3"("start path"=w454, "prompt"="Save image", "button label"="Save", "error in"=w446, "pattern (all files)"=".png", "pattern label"="PNG") -> ("selected path"=w456:path, "error out"=w448:errorcluster)  [unwired: 6 in, 2 out]
                  n154 = call-poly "IMAQ Write File 2"("error in (no error)"=w448, "File Path"=w456, "Image"=w445) -> ("error out"=w447:errorcluster)  [unwired: 7 in, 1 out]
                }
              }
              n155 = Array Size(array=w432) -> (size(s)=w431:i32)
              n156 = Decrement(x=w431) -> (x-1=w430:i32)
              n157 = Index Array(array=w432, index=w430) -> (element=w433:u32)
              n158 = call "IMAQ UserLookup 2"("Image Src"=w427, "Lookup Table"=i32[] []) -> ("Image Dst Out"=w426:T1)  [unwired: 5 in, 1 out]
            }
            frame True {
              n159 = call <vilib>:"IMAQdx Snap.vi"("error in"=w472, "Image In"=w471, "Session In"=w470) -> ("error out"=w475:errorcluster, "Image Out"=w467:T1, "Session Out"=w474:T4)  [unwired: 6 in]
              n160 = call "IMAQ ColorHistograph"("Image Src"=w467) -> ("Red or Hue Histogram Graph"=w466:T3, "Green or Sat Histogram Graph"=w465:T3, "Blue or Luma or Val or Inten Histogram Graph"=w464:T3)  [unwired: 5 in, 1 out]
              n161 = Compound Arithmetic op=ADD(w466, w465, w464) -> (w463:T3)
              n162 = Unbundle(w463) -> ("Histogram"=w461:u32[])  [unwired: 2 out]
              n163 = case shown="True" w473 {
                tunnel: [w477 w487] -> w476
                tunnel: w467 -> [_ w478]
                tunnel: w475 -> [w477 w479]
                frame False {
                }
                frame True {
                  n164 = property on="path" class="Path"() -> ("Value"=w486:path)  [unwired: 2 in, 2 out]
                  n165 = Build Path(base path=w486, name or relative path="Images") -> (appended path=w485:path)
                  n166 = call "File Dialog2"("start path"=w485, "prompt"="Save image", "button label"="Save", "error in"=w479, "pattern (all files)"=".png", "pattern label"="PNG") -> ("selected path"=w489:path, "error out"=w488:errorcluster)  [unwired: 6 in, 2 out]
                  n167 = call-poly "IMAQ Write File 2"("error in (no error)"=w488, "File Path"=w489, "Image"=w478) -> ("error out"=w487:errorcluster)  [unwired: 7 in, 1 out]
                }
              }
              n168 = Array Size(array=w461) -> (size(s)=w460:i32)
              n169 = Decrement(x=w460) -> (x-1=w459:i32)
              n170 = Index Array(array=w461, index=w459) -> (element=w462:u32)
            }
          }
          "Image" <- w253
          "Histograph" <- w252
          "# Sat. Pixels" <- w251
          n171 = case shown="No Error" w264 {
            tunnel: [FALSE ("true") w491] -> w265
            frame No Error {
            }
            frame Error {
              n172 = property on="path" class="Path"() -> ("Value"=w495:path)  [unwired: 2 in, 2 out]
              n173 = Build Path(base path=w495, name or relative path="SupportFiles\\TestPatterns\\test_patern.bmp") -> (appended path=w494:path)
              n174 = property on="selected path 2" class="Path"("Value"=w494) -> ()  [unwired: 2 in, 2 out]
              n175 = One Button Dialog(message="Do NOT exist the selected image. Please, chose another file to diplay on SLM2") -> (true=w491:bool)  [unwired: 1 in]
            }
          }
          n176 = case shown="Error" w262 {
            tunnel: [FALSE ("true") w499] -> w266
            frame No Error {
            }
            frame Error {
              n177 = property on="path" class="Path"() -> ("Value"=w497:path)  [unwired: 2 in, 2 out]
              n178 = Build Path(base path=w497, name or relative path="SupportFiles\\TestPatterns\\test_patern.bmp") -> (appended path=w500:path)
              n179 = property on="selected path" class="Path"("Value"=w500) -> ()  [unwired: 2 in, 2 out]
              n180 = One Button Dialog(message="Do NOT exist the selected image. Please, chose another file to diplay on SLM1") -> (true=w499:bool)  [unwired: 1 in]
            }
          }
          n181 = property on="Histograph" class="WFGraph (strict)"("XScale.Maximum"=w250) -> ()  [unwired: 2 in, 2 out]
          n182 = local read "Set Current at:"() -> (w278:sgl)
          n183 = invoke class="APTLaser" method="ReadLaserCurrent"(reference=w281, error in=w247, "pfCurrent"=w278) -> (reference out=w280:refnum<k7>, error out=w246:errorcluster, "pfCurrent"=w276:sgl)  [unwired: 1 in, 1 out]
          n184 = property on="Histograph" class="WFGraph (strict)"("YScale.Maximum"=w249) -> ()  [unwired: 2 in, 2 out]
          n185 = Multiply(x=w276, y=sgl 0.2) -> (x*y=w279:sgl)
          n186 = Add(x=w279, y=sgl -10.0) -> (x+y=w258:sgl)
          "Power" <- w258
          n187 = Greater?(x=w258, y=sgl 7.0) -> (0:w287:bool)
          n188 = case shown="True" w287 {
            tunnel: w258 -> [w371 w375]
            tunnel: [w372 w378] -> w286
            frame False {
              n189 = Greater?(x=w371, y=sgl 2.0) -> (0:w369:bool)
              n190 = case shown="True" w369 {
                tunnel: [u32 1985280 u32 6618880] -> w372
                frame False {
                }
                frame True {
                }
              }
            }
            frame True {
              n191 = Greater?(x=w375, y=13.0) -> (0:w376:bool)
              n192 = case shown="True" w376 {
                tunnel: [u32 16749164 u32 16711680] -> w378
                tunnel: w375 -> [_ w383]
                frame False {
                }
                frame True {
                  n193 = Greater?(x=w383, y=sgl 15.0) -> (0:w381:bool)
                  n194 = property on="Color Box" class="ColBox"("Blinking"=w381) -> ()  [unwired: 2 in, 2 out]
                }
              }
            }
          }
          "Color Box" <- w286
          n195 = Compound Arithmetic op=OR(w266, w265, w260, w259) -> (w294:bool)
          n196 = call "IMAQ WindClose"("Close All Windows (False)"=w294) -> ()  [unwired: 5 in, 1 out]
        }
        "selected path" <- w224
        "selected path 2" <- w223
      }
    }
    n197 = call "IMAQ WindClose"("Close All Windows (False)"=w50) -> ()  [unwired: 5 in, 1 out]
    n198 = call "IMAQ Dispose"("All Images? (No)"=w50) -> ()  [unwired: 5 in, 1 out]
  }
  "error out" <- w33
  "error out 2" <- w32
  "error out 6" <- w1
  n199 = Not(x=w38) -> (.not. x?=w26:bool)
  n200 = property on="Power" class="Knob (strict)"("Value"=w21) -> ()  [unwired: 2 in, 2 out]
  n201 = invoke class="APTLaser" method="DisableOutput"(reference=w28, error in=w6) -> (reference out=w27:refnum<k7>, error out=w5:errorcluster)  [unwired: 1 in, 1 out]
  n202 = call <vilib>:"IMAQdx Close Camera.vi"("error in"=w13, "Session In"=w14) -> ("error out"=→"error out 4":errorcluster)  [unwired: 9 in]
  n203 = call <vilib>:"IMAQdx Close Camera.vi"("error in"=w15, "Session In"=w16) -> ("error out"=→"error out 3":errorcluster)  [unwired: 9 in]
  n204 = property on="Parada Total" class="Bool (strict)"("Value"=w26) -> ()  [unwired: 2 in, 2 out]
  n205 = property on="LaserON" class="Bool (strict)"("Value"=w26) -> ()  [unwired: 2 in, 2 out]
  n206 = property on="Color Box" class="ColBox"("Value"=w22) -> ()  [unwired: 2 in, 2 out]
  n207 = invoke class="APTLaser" method="StopCtrl"(reference=w27, error in=w5) -> (error out=→"error out 5":errorcluster)  [unwired: 1 in, 2 out]
